vi "Close Test Log.vi"(8 "error in (no error)":errorcluster, 11 "Model in":refnum<class "Model.lvclass">) -> (0 "error out":errorcluster, 3 "Model out":refnum<class "Model.lvclass">)   [LabVIEW 2015, in "Model.lvclass"]
uses:
  Model.lvclass
  Model.lvclass/Model.ctl
  Test Log/Test Log/Test Log.lvclass
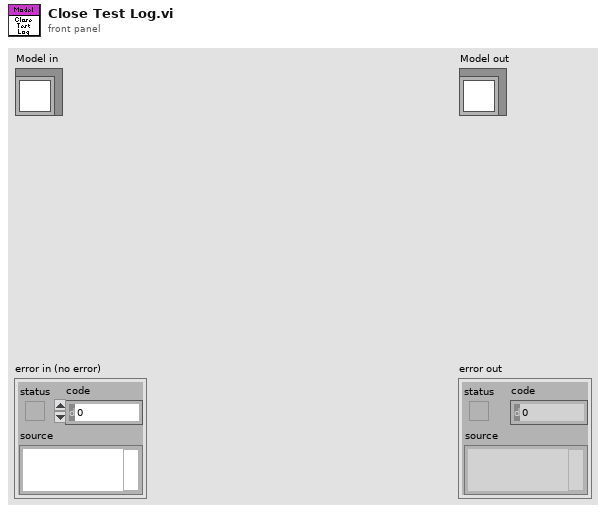
[diagram p1: front panel]
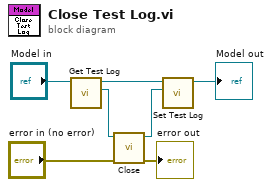
[diagram p0: block diagram]
diagram:
  n1 = call "Get Test Log.vi"("Model in"="Model in") -> ("ITestLog.lvclass"=w6:refnum<class "Test Log.lvclass">, "Model out"=w5:refnum<class "Model.lvclass">)  [unwired: 9 in]
  n2 = call-dynamic "Close.vi"("error in (no error)"="error in (no error)", "Test Log in"=w6) -> ("error out"=→"error out":errorcluster, "Test Log out"=w7:refnum<class "Test Log.lvclass">)  [unwired: 8 in]
  n3 = call "Set Test Log.vi"("ITestLog.lvclass"=w7, "Model in"=w5) -> ("Model out"=→"Model out":refnum<class "Model.lvclass">)  [unwired: 9 in]
